vi "Read VI reference.vi"(8 "error in (no error)":errorcluster, 11 "UI Load SubPanel Display in":refnum<class "UI Load SubPanel Display.lvclass">) -> (0 "error out":errorcluster, 2 "VI reference":refnum<vi>, 3 "UI Load SubPanel Display out":refnum<class "UI Load SubPanel Display.lvclass">)   [LabVIEW 2011, in "UI Load SubPanel Display.lvclass"]
uses:
  UI Load SubPanel Display.lvclass
  UI Load SubPanel Display.lvclass/UI Load SubPanel Display.ctl
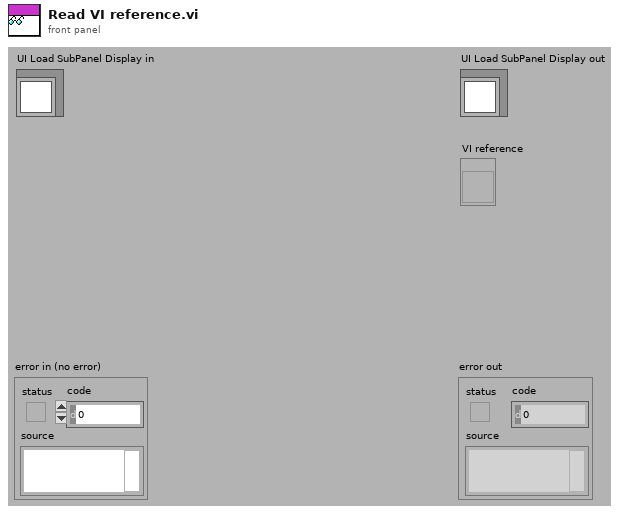
[diagram p1: front panel]
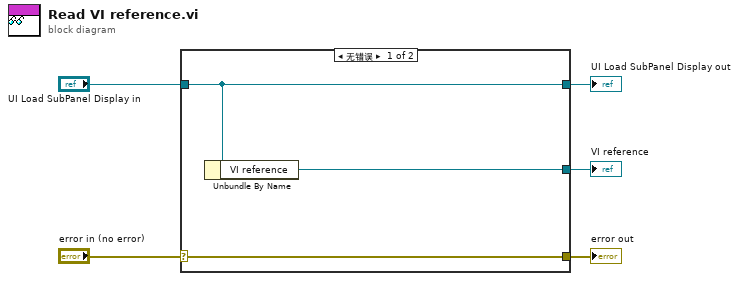
[diagram p0: block diagram]
diagram:
  n1 = case shown="无错误" "error in (no error)" {
    selector: "error in (no error)" -> [w8 w9]
    tunnel: [w8 w9] -> w4
    tunnel: [w7 w10] -> w2
    tunnel: "UI Load SubPanel Display in" -> [w7 w10]
    tunnel: [w6 _] -> w1
    frame No Error {
      n2 = Unbundle By Name(w7) -> ("VI reference"=w6:refnum<vi>)
    }
    frame Error {
    }
  }
  "error out" <- w4
  "UI Load SubPanel Display out" <- w2
  "VI reference" <- w1
